vi "SetEnvCover.vi"(7 "LabVIEW Web Service Request":refnum<class "Web Request.lvclass">, 11 "cov":string) -> (3 "result":string)   [LabVIEW 2016]
uses:
  <vilib>/wsapi/Web Request.lvclass
  controls/SwitchStates.ctl
  controls/MotorSetStates.ctl
  controls/RT-Variables.lvlib
panel:
  # "Use the Web Service Request input terminal to call the VIs on the Web Services palette. Do not remove it from the connector pane unless you don't need access to the palette."
  # "Each additional control wired to the connector pane will be available as an input in the URL. To include an indicator in terminal-mode output (the default setting), it must also be wired to the connector pane."
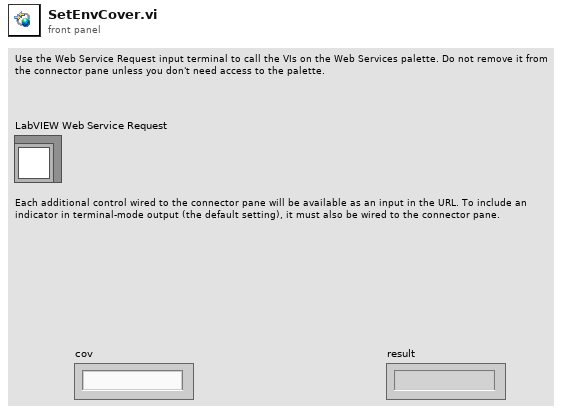
[diagram p1: front panel]
types:
  T1 = typedef "RT-Variables.lvlib/SwitchStates.ctl" = enum16{"Off", "Local", "Remote"}
  T2 = typedef "RT-Variables.lvlib/MotorSetStates.ctl" = enum16{"Open", "Close"}
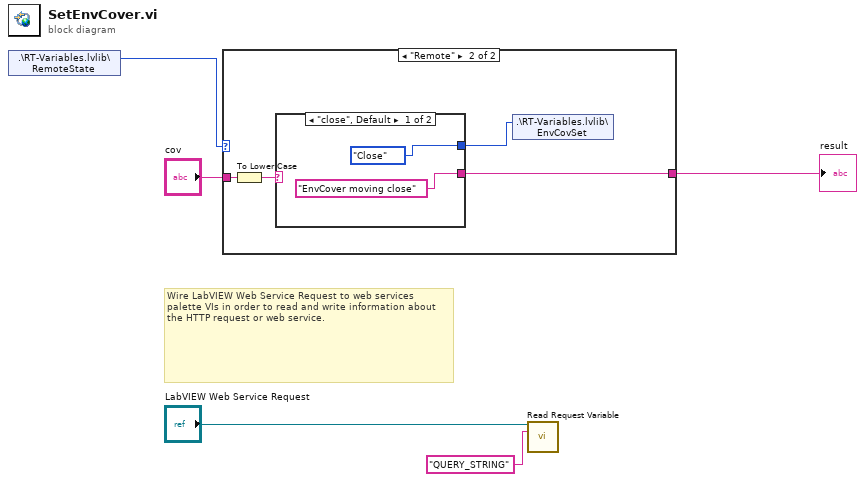
[diagram p0: block diagram]
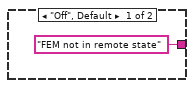
[diagram p2: hidden frame]
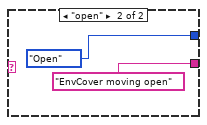
[diagram p3: hidden frame]
diagram:
  # "Wire LabVIEW Web Service Request to web services palette VIs in order to read and write information about the HTTP request or web service."
  n1 = shared-variable ".\\RT-Variables.lvlib\\RemoteState"() -> (w2:T1)  [unwired: 1 in, 1 out]
  n2 = case shown="\"Remote\"" w2 {
    tunnel: "cov" -> [_ w10]
    tunnel: ["FEM not in remote state" w8] -> w1
    frame "Off", Default {
    }
    frame "Remote" {
      n3 = To Lower Case(string=w10) -> (all lower case string=w9:string)
      n4 = case shown="\"close\", Default" w9 {
        tunnel: ["EnvCover moving close" "EnvCover moving open"] -> w8
        tunnel: [MotorSetStates."Close" ("EnvCoverPos") MotorSetStates."Open" ("EnvCoverPos")] -> w7
        frame "close", Default {
        }
        frame "open" {
        }
      }
      n5 = shared-variable ".\\RT-Variables.lvlib\\EnvCovSet"(w7) -> ()  [unwired: 1 in, 1 out]
    }
  }
  "result" <- w1
  n6 = call <vilib>:"Read Request Variable.vi"("LabVIEW Web Service Request"="LabVIEW Web Service Request", "variable name"="QUERY_STRING") -> ()  [unwired: 11 in, 3 out]
